vi "Configure Source to Sequence-Single.vi"(8 "error in":errorcluster, 11 "Source to seq config - Single":T1={"Source channel name"="", "Source out"="", "Source sweep values"=[], "Load sweep points"=0, "Source output function"=1006, "Source transient response"=1038, "Source voltage/current gain bandwidth"=0.0, "Source voltage/current compensation frequency"=0.0, "Source voltage/current pole-zero ratio"=0.0, "Source aperture time"=0.0, "Source source delay"=0.0} {"Source transient response" items=["Slow"=1041, "Normal"=1038, "Fast"=1039, "Custom"=1042]; "Source output function" items=["DC Voltage"=1006, "DC Current"=1007, "Pulse Voltage"=1049, "Pulse Current"=1050]; "Source sweep values" format="%#_13g"}) -> (0 "error out":errorcluster, 2 "Source channel name":string, 3 "instrument handle out":refnum<k15>)   [LabVIEW 2021]
doc: "This VI create source sequence for signle configuration of source"
uses:
  controls/Source to Sequence Config-Single.ctl
  <instrlib>/niDCPower/nidcpower.llb/niDCPower Source Mode.ctl
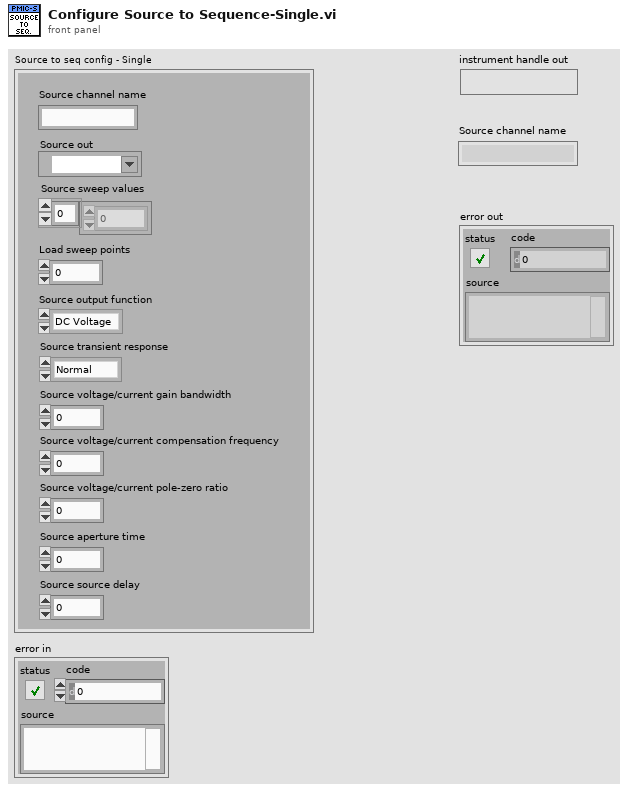
[diagram p1: front panel]
types:
  T1 = typedef "Source to Sequence Config-Single.ctl" = cluster{"Source channel name":string, "Source out":refnum<k15>, "Source sweep values":dbl[], "Load sweep points":i32, "Source output function":i32, "Source transient response":i32, "Source voltage/current gain bandwidth":dbl, "Source voltage/current compensation frequency":dbl, "Source voltage/current pole-zero ratio":dbl, "Source aperture time":dbl, "Source source delay":dbl}
  T2 = typedef "niDCPower Source Mode.ctl" = i32
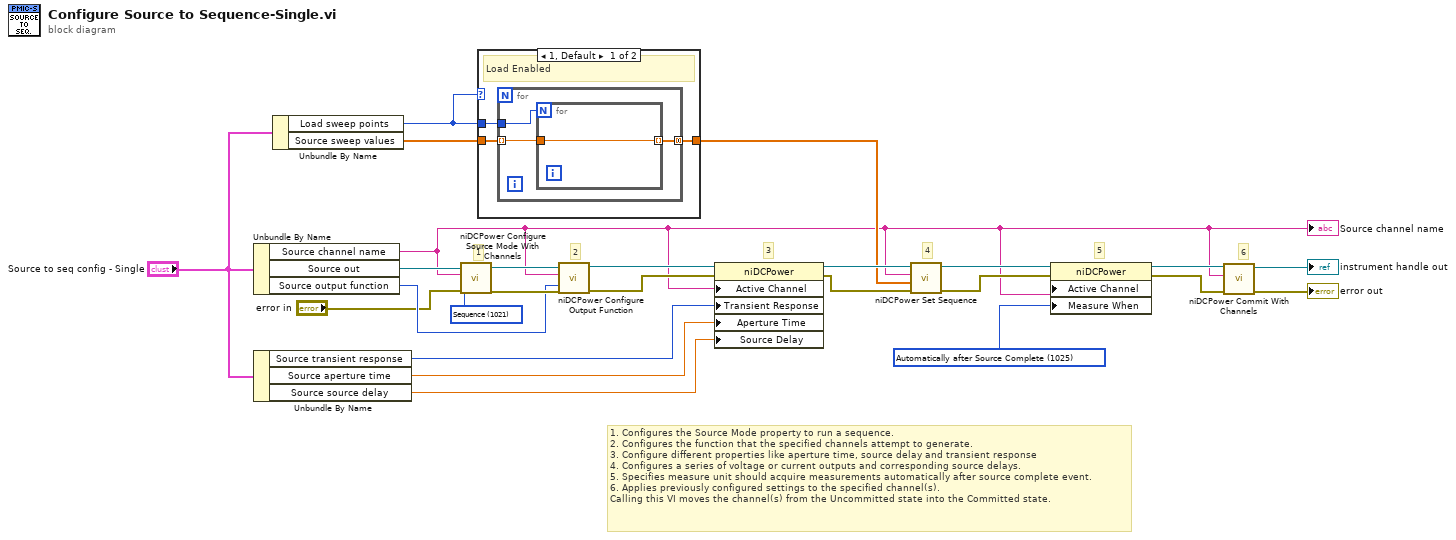
[diagram p0: block diagram]
diagram:
  w6 = T2 1021 items=["Single Point"=1020, "Sequence"=1021] ("source mode")
  w10 = 1025 items=["Automatically after Source Complete"=1025, "On Demand"=1026, "On Measure Trigger"=1027] ("Measurement:Advanced:Measure When")
  # "6"
  # "5"
  # "4"
  # "3"
  # "2"
  # "1"
  # "1. Configures the Source Mode property to run a sequence.\n2. Configures the function that the specified channels attempt to generate.\n3. Configure different properties like aperture time, source delay and transient response\n4. Configures a series of voltage or current outputs and corresponding source delays. \n5. Specifies measure unit should acquire measurements automatically after source complete event.\n6. Applies previously configured settings to the specified channel(s).\nCalling this VI moves the channel(s) from the Uncommitted state into the Committed state."
  n1 = Unbundle By Name("Source to seq config - Single") -> ("Source channel name"=w5:string, "Source out"=w25:refnum<k15>, "Source output function"=w23:i32)
  "Source channel name" <- w5
  n2 = Unbundle By Name("Source to seq config - Single") -> ("Source transient response"=w18:i32, "Source aperture time"=w19:dbl, "Source source delay"=w2:dbl)
  n3 = Unbundle By Name("Source to seq config - Single") -> ("Load sweep points"=w14:i32, "Source sweep values"=w13:dbl[])
  n4 = call <instrlib>:"niDCPower Configure Source Mode With Channels.vi"("error in (no error)"="error in", "source mode"=w6, "channel name"=w5, "instrument handle"=w25) -> ("error out"=w24:errorcluster, "instrument handle out"=w22:refnum<k15>)  [unwired: 6 in]
  n5 = case shown="1, Default" w14 {
    tunnel: w14 -> [w28 _]
    tunnel: w13 -> [w27 w33]
    tunnel: [w26 w33] -> w12
    frame 1, Default {
      # "Load Enabled"
      n6 = for {
        tunnel: w28 -> [w31]
        tunnel: w27 -> [w30] mode=indexing
        tunnel: [w29] -> w26 mode=concatenating
        n7 = for {
          N: w31 -> [_]
          tunnel: w30 -> [w32]
          tunnel: [w32] -> w29 mode=indexing
        }
      }
    }
    frame 0 {
      # "Load Disab;ed"
    }
  }
  n8 = call <instrlib>:"niDCPower Configure Output Function.vi"("error in (no error)"=w24, "output function"=w23, "channel name"=w5, "instrument handle"=w22) -> ("error out"=w20:errorcluster, "instrument handle out"=w21:refnum<k15>)  [unwired: 6 in]
  n9 = property class="niDCPower"(reference=w21, error in=w20, "Active Channel"=w5, "Transient Response"=w18, "Aperture Time"=w19, "Source Delay"=w2) -> (reference out=w17:refnum<k15>, error out=w16:errorcluster)
  n10 = call <instrlib>:"niDCPower Set Sequence.vi"("error in (no error)"=w16, "values"=w12, "channel name"=w5, "instrument handle"=w17) -> ("error out"=w9:errorcluster, "instrument handle out"=w11:refnum<k15>)  [unwired: 6 in]
  n11 = property class="niDCPower"(reference=w11, error in=w9, "Active Channel"=w5, "Measure When"=w10) -> (reference out=w8:refnum<k15>, error out=w7:errorcluster)
  n12 = call <instrlib>:"niDCPower Commit With Channels.vi"("error in (no error)"=w7, "channel name"=w5, "instrument handle"=w8) -> ("error out"=→"error out":errorcluster, "instrument handle out"=→"instrument handle out":refnum<k15>)  [unwired: 7 in]
